vi "Timestamp Now if Default.vi"(10 "timestamp in":timestamp format="%<%x %.3X>T") -> (2 "timestamp out":timestamp format="%<%x %.3X>T")   [LabVIEW 2020, in "g-sugar.lvlib"]
doc: "If the input timestamp is default, returns the current timestamp, else passes the input timestamp."
uses:
  g-sugar.lvlib
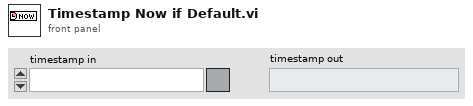
[diagram p1: front panel]
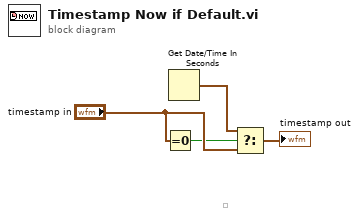
[diagram p0: block diagram]
diagram:
  n1 = Equal To 0?(x="timestamp in") -> (x = 0?=w1:bool)
  n2 = Get Date/Time In Seconds() -> (seconds since 1Jan1904=w2:timestamp)
  n3 = Select(t=w2, s=w1, f="timestamp in") -> (s? t:f=→"timestamp out":timestamp)
